vi "tvi_arx_ni9234_global.vi"() -> ()   [LabVIEW 2012]
panel:
  out "standstill boolean":bool
  out "1 stride boolean":bool
  out "main loop boolen":bool
  out "step-interval":dbl
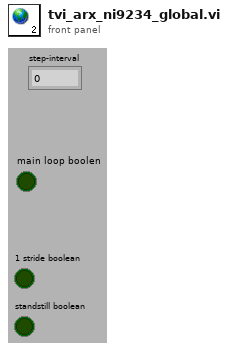
[diagram p1: front panel]
diagram:
